vi "Freq_amp_Corr.vi"(10 "Input STFT":dbl[][](array[numeric])) -> (2 "Output STFT":dbl[][](array[numeric]))   [LabVIEW 2014, in "Melody Extraction.lvlib"]
uses:
  Melody Extraction.lvlib
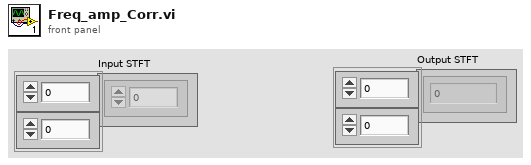
[diagram p1: front panel]
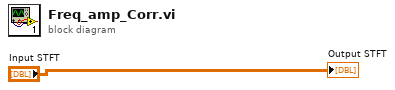
[diagram p0: block diagram]
diagram:
  "Output STFT" <- "Input STFT"
